vi "writeToXML.vi"(8 "error in (no error)":errorcluster, 10 "ClassLabel":string, 11 "OffsetStatus in":refnum<class "OffsetStatus.lvclass">) -> (0 "error out":errorcluster, 2 "XML out":string, 3 "OffsetStatus out":refnum<class "OffsetStatus.lvclass">)   [LabVIEW 2022 SP3, in "TCSDataDefinitions.lvlib" / "TCSPublicStatus.lvlib" / "OffsetStatus.lvclass"]
uses:
  OffsetStatus.lvclass
  <userlib>/Common/UnitsAndXML/FlattenItemWithUnitToXML/FlattenTimeToXML/TimeUnit.ctl
  <userlib>/Common/UnitsAndXML/FlattenItemWithUnitToXML/FlattenPlaneAngleToXML/PlaneAngleUnit.ctl
  OffsetStatus.lvclass/OffsetStatus.ctl
  <userlib>/Common/UnitsAndXML/UnitsAndXML.lvlib
  <userlib>/Common/XML/XMLGenerator/XMLGenerator.lvclass
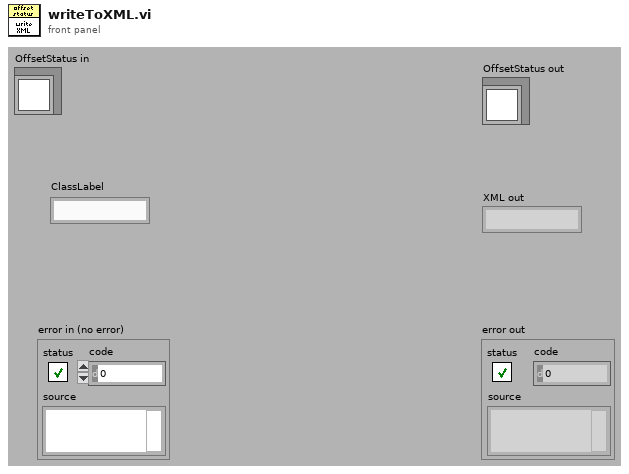
[diagram p1: front panel]
types:
  T1 = typedef "UnitsAndXML.lvlib/PlaneAngleUnit.ctl" = enum16{"rad", "deg", "'", "\""}
  T2 = typedef "UnitsAndXML.lvlib/TimeUnit.ctl" = enum16{"s", "d", "h", "min", "a"}
  T3 = typedef "TCSDataDefinitions.lvlib/TCSCommand.lvlib/OffsetCommands.lvlib/OffsetType.ctl" = enum16{"SIMPLE", "TPLANE", "PA"}
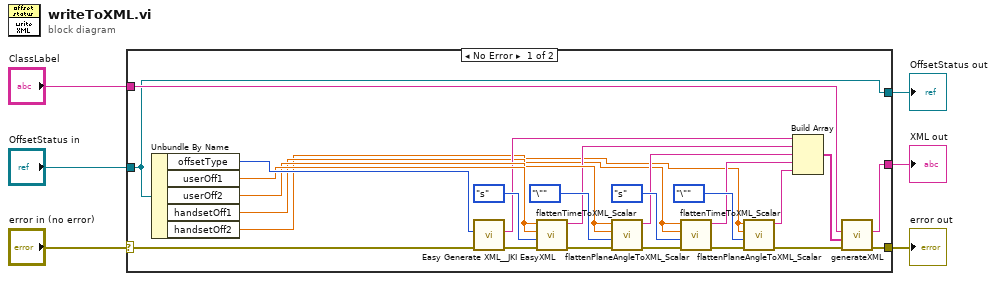
[diagram p0: block diagram]
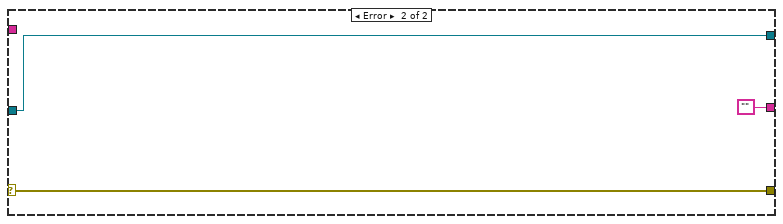
[diagram p2: hidden frame]
diagram:
  n1 = case shown="No Error" "error in (no error)" {
    selector: "error in (no error)" -> [w7 w34]
    tunnel: [w29 w34] -> w5
    tunnel: [w26 w33] -> w1
    tunnel: "OffsetStatus in" -> [w26 w33]
    tunnel: "ClassLabel" -> [w28 _]
    tunnel: [w27 ""] -> w3
    frame No Error {
      n2 = Unbundle By Name(w26) -> ("offsetType"=w31:T3, "userOff1"=w19:dbl[unit], "userOff2"=w18:dbl[unit], "handsetOff1"=w9:dbl[unit], "handsetOff2"=w8:dbl[unit])
      n3 = call <vilib>:"Easy Generate XML__JKI EasyXML.vi"("error in (no error)"=w7, "LabVIEW Data"=w31) -> ("error out"=w17:errorcluster, "XML String"=w14:string)  [unwired: 8 in]
      n4 = call <userlib>:"flattenTimeToXML_Scalar.vi"("error in (no error)"=w17, "timeUnitInXML"=TimeUnit."s", "timeAgain"=w19, "time"=w19) -> ("error out"=w23:errorcluster, "xmlString"=w13:string)  [unwired: 6 in]
      n5 = call <userlib>:"flattenPlaneAngleToXML_Scalar.vi"("error in (no error)"=w23, "planeAngleUnitInXML"=PlaneAngleUnit."\"", "planeAngleAgain"=w18, "planeAngle"=w18) -> ("error out"=w16:errorcluster, "xmlString"=w12:string)  [unwired: 6 in]
      n6 = call <userlib>:"flattenTimeToXML_Scalar.vi"("error in (no error)"=w16, "timeUnitInXML"=TimeUnit."s", "timeAgain"=w9, "time"=w9) -> ("error out"=w20:errorcluster, "xmlString"=w11:string)  [unwired: 6 in]
      n7 = call <userlib>:"flattenPlaneAngleToXML_Scalar.vi"("error in (no error)"=w20, "planeAngleUnitInXML"=PlaneAngleUnit."\"", "planeAngleAgain"=w8, "planeAngle"=w8) -> ("error out"=w15:errorcluster, "xmlString"=w10:string)  [unwired: 6 in]
      n8 = Build Array(w14, w13, w12, w11, w10) -> (w30:string[])
      n9 = call <userlib>:"generateXML.vi"("error in"=w15, "childrenXML"=w30, "elementName"=w28) -> ("error out"=w29:errorcluster, "XML out"=w27:string)  [unwired: 6 in, 1 out]
    }
    frame Error {
    }
  }
  "error out" <- w5
  "XML out" <- w3
  "OffsetStatus out" <- w1
